vi "OP400ZP_VGConf.vi"() -> ()   [LabVIEW 2020]
panel:
  out "Max":dbl
  out "VCellMax70":dbl
  out "VCellMin70":dbl
  out "VCellMax30":dbl
  out "VCellMin30":dbl
  out "DeltaV":dbl
  out "ZEN79TENS":dbl
  out "ZEN84":dbl
  out "ZEN82":dbl
  out "ZEN79":dbl
  out "ZEN77":dbl
  out "ZEN74":dbl
  out "DeltaT":dbl
  out "TusineMax":dbl
  out "TusineMin":dbl
  out "TCellMax":dbl
  out "TCellMin":dbl
  out "ZEN79min30":dbl
  out "ZEN77max30":dbl
  out "ZEN84min70":dbl
  out "ZEN84max70":dbl
  out "ZEN84min30":dbl
  out "ZEN84max30":dbl
  out "ZEN82min70":dbl
  out "ZEN82max70":dbl
  out "ZEN82min30":dbl
  out "ZEN82max30":dbl
  out "ZEN79min70":dbl
  out "ZEN77max70":dbl
  out "ZEN79max70":dbl
  out "ZEN77min30":dbl
  out "ZEN79max30":dbl
  out "ZEN74min70":dbl
  out "ZEN77min70":dbl
  out "ZEN74max70":dbl
  out "ZEN74min30":dbl
  out "ZEN74max30":dbl
  out "Rmin":dbl
  out "Rmax":dbl
  in  "3562":string
  in  "MX5060":string
  in  "ST5520":string
  # "///////Config SOC 70%\n\n[EQUIPEMENT]\n3562 = HIOKI,BT3562A,0,V2.01\n\n[Conti]\nRmax = 40\nRmin = 1\n\n[OCV]\nZEN74max30 = 621\nZEN74min30 = 588\nZEN74max70 = 672\nZEN74min70 = 634\nZEN77max30 = 643\nZEN77min30 = 609\nZEN77max70 = 696\nZEN77min70 = 656\nZEN79max30 = 666\nZEN79min30 = 630\nZEN79max70 = 720\nZEN79min70 = 679\nZEN82max30 = 689\nZEN82min30 = 651\nZEN82max70 = 744\nZEN82min70 = 701\nZEN84max30 = 711\nZEN84min30 = 672\nZEN84max70 = 768\nZEN84min70 = 724\n\n[DataDyn]\nTCellMin = 16\nTCellMax = 32\nTusineMin = 16\nTusineMax = 32\nDeltaT = 3\nDeltaV = 30\n\nVCellMin30 = 3500\nVCellMax30 = 3700\nVCellMin70 = 3800\nVCellMax70 = 4000\n\n\n[PN]\n00083338 = ZEN77\n00084480 = ZEN77\n00084997 = ZEN84\n\n[Sealing]\nMax = 200\n\n[NbModule]\nZEN74 = 28\nZEN77 = 29\nZEN79 = 30\nZEN82 = 31\nZEN84 = 32"
  # "EQUIPEMENTS"
  # "Conti"
  # "Sealing"
  # "OCV"
  # "DataDyn"
  # "NbModule"
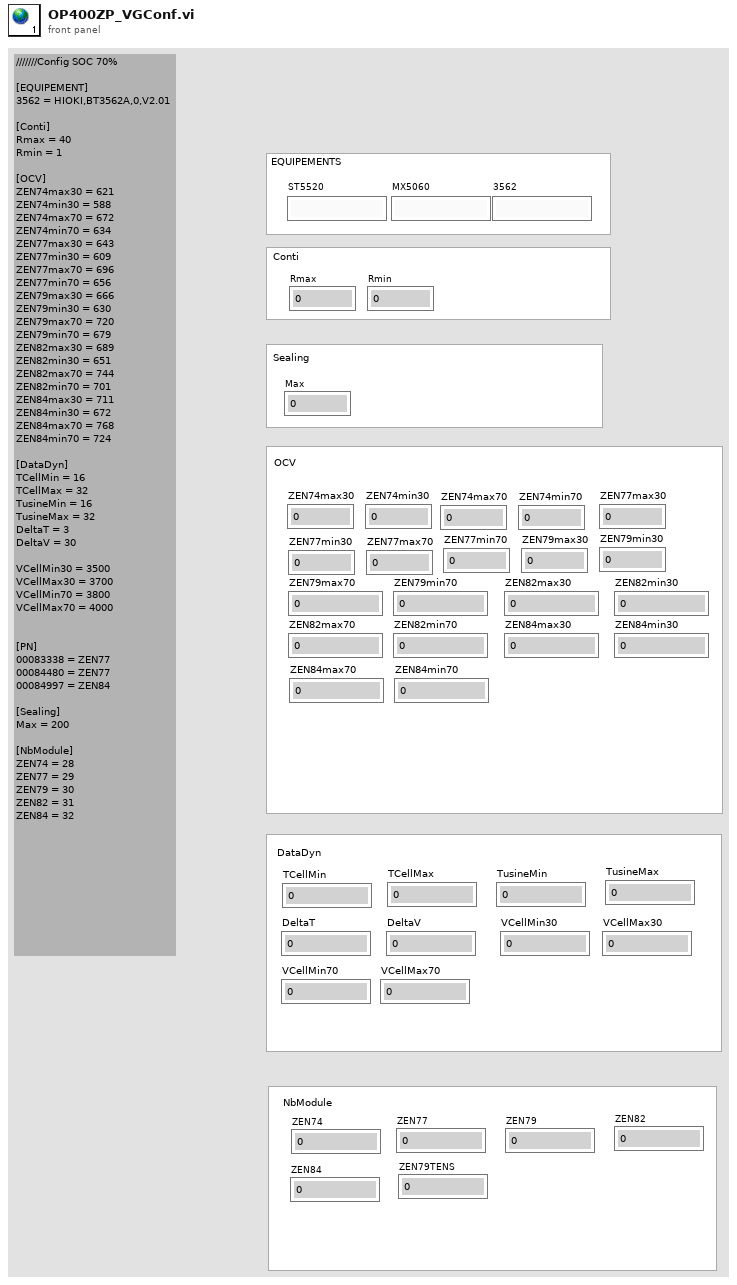
[diagram p1: front panel]
diagram:
